vi "RunVI.vi"(0 "VI Reference In":refnum<vi>, 5 "Wait Until Done (F)":bool, 7 "Auto Dispose Reference (F)":bool, 11 "error in":errorcluster) -> (4 "VI Reference Out":refnum<vi>, 15 "error out":errorcluster)   [LabVIEW 2016, in "Drona.lvlib"]
doc: "Runs the VI, given the VI reference."
uses:
  Drona.lvlib
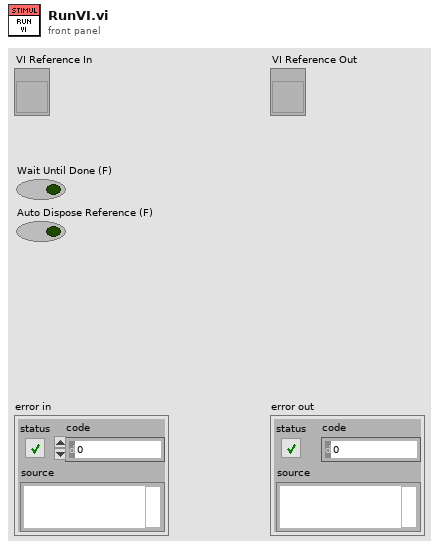
[diagram p1: front panel]
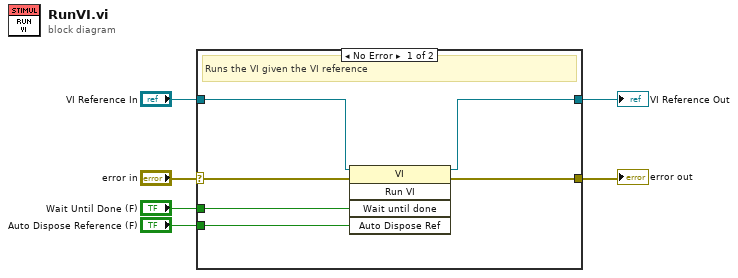
[diagram p0: block diagram]
diagram:
  n1 = case shown="No Error" "error in" {
    selector: "error in" -> [w7 w14]
    tunnel: "VI Reference In" -> [w11 w13]
    tunnel: [w10 w13] -> w4
    tunnel: [w12 w14] -> w3
    tunnel: "Wait Until Done (F)" -> [w9 _]
    tunnel: "Auto Dispose Reference (F)" -> [w8 _]
    frame No Error {
      # "Runs the VI given the VI reference"
      n2 = invoke on="Invoke Node" class="VI" method="Run VI"(reference=w11, error in=w7, "Wait until done"=w9, "Auto Dispose Ref"=w8) -> (reference out=w10:refnum<vi>, error out=w12:errorcluster)  [unwired: 1 in, 3 out]
    }
    frame Error {
    }
  }
  "error out" <- w3
  "VI Reference Out" <- w4
